vi "CloseMaster.vi"(2 "error in (no error)":errorcluster) -> (0 "error out":errorcluster)   [LabVIEW 2015]
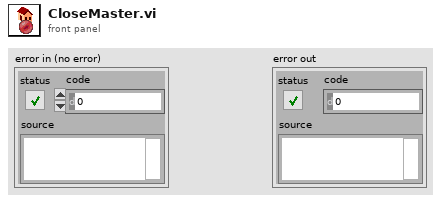
[diagram p1: front panel]
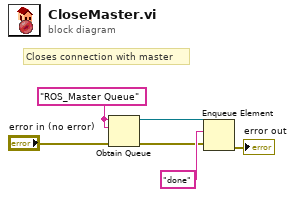
[diagram p0: block diagram]
diagram:
  w4 = "ROS_Master Queue" ("name (unnamed)")
  # "Closes connection with master"
  n1 = Obtain Queue(name (unnamed)=w4, element data type=w4, error in (no error)="error in (no error)") -> (queue out=w6:refnum<queue>, error out=w1:errorcluster)  [unwired: 2 in, 1 out]
  n2 = Enqueue Element(queue=w6, element="done", error in (no error)=w1) -> (error out=→"error out":errorcluster)  [unwired: 1 in, 2 out]
